vi "test-diff-drive-constraints.vi"() -> (3 "Test Passed":bool)   [LabVIEW 2019]
uses:
  <vilib>/Rock Robotics/WPI/ThirdParty/JAS_Junk/TrajLib/POSE2D.ctl
  <vilib>/Rock Robotics/WPI/ThirdParty/JAS_Junk/TrajLib/TRANSLATION2D.ctl
  <vilib>/Rock Robotics/WPI/ThirdParty/JAS_Junk/TrajLib/ROTATION2D.ctl
  <vilib>/Rock Robotics/SystemInterfaces/NetworkCommunication/NetComm_UsageReport_report.vi
  <vilib>/Rock Robotics/WPI/ThirdParty/JAS_Junk/TrajLib/DiffDriveKinematicsConstraint_New.vi
  <vilib>/Rock Robotics/WPI/ThirdParty/JAS_Junk/TrajLib/CentripetalAccelConstraint_New.vi
  <vilib>/Rock Robotics/WPI/ThirdParty/JAS_Junk/TrajLib/Util_LibraryGlobals.vi
  <vilib>/Rock Robotics/WPI/ThirdParty/JAS_Junk/TrajLib/Trajectory_Library.lvlib
panel:
  in  "Cent Feet Per Sec^2 2":dbl=12.0 format="%#_13g"
  out "Accel Exceeded":bool
  out "Acceleration":dbl[][](graph)
  out "Velocity":dbl[][](graph)
  out "Max Accel":dbl
  out "Max Ya":dbl
  out "max Xx":dbl
  in  "Feet/Sec":dbl=12.0 format="%#_13g"
  in  "Feet Per Sec^2":dbl=12.0 format="%#_13g"
  out "Max Speed":dbl
  out "Max Y vel":dbl
  out "max X vel":dbl
  out "XY Graph":cluster{dbl[], dbl[]}[](graph)
  out "Waypoints":T1[](array[typedef]) {"ROTATION"."SIN" format="%13.4f"; "ROTATION"."COS" format="%13.4f"; "ROTATION"."VALUE" format="%13.4f"; "TRANSLATION"."Y" format="%14.3f"; "TRANSLATION"."X" format="%14.3f"}
  out "TotalTImeSecs":dbl
  out "Speed Exceeded":bool
  out "error out":errorcluster
  # "9.1"
  # "5.7"
  # "9.55"
  # "6.59"
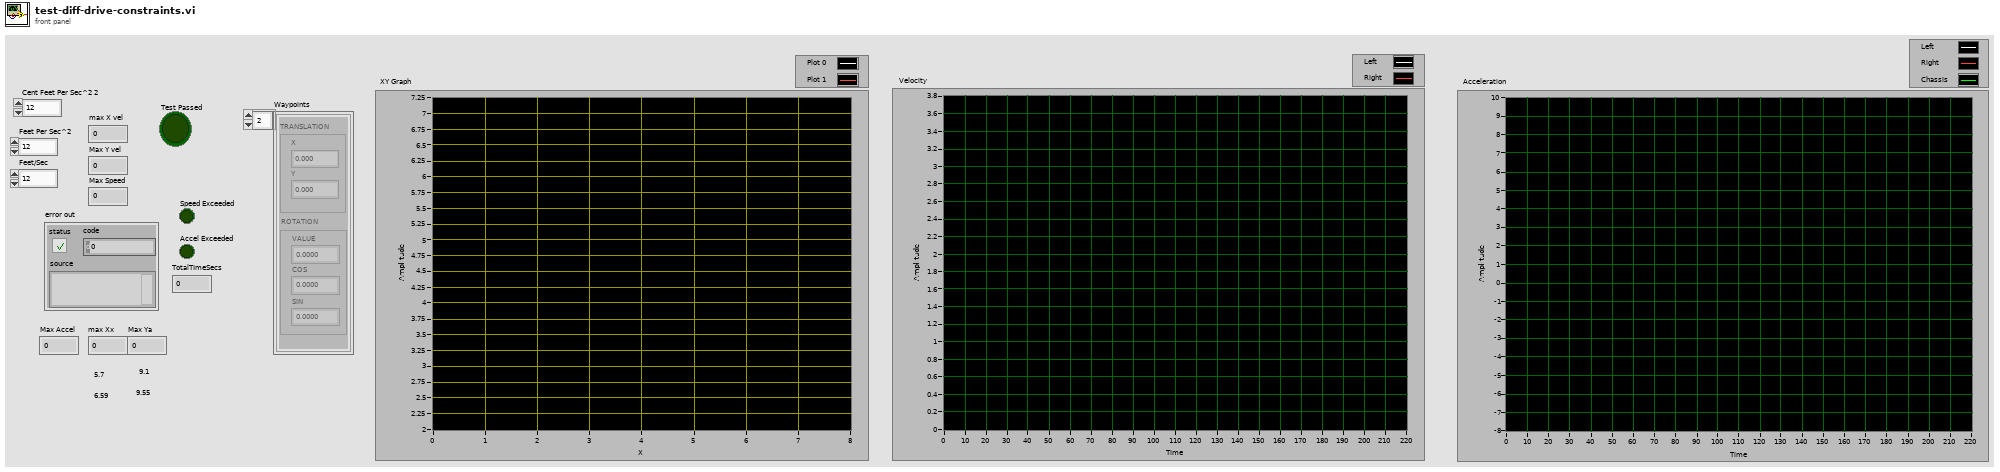
[diagram p1: front panel]
types:
  T1 = typedef "Trajectory_Library.lvlib/POSE2D.ctl" = cluster{"TRANSLATION":T2, "ROTATION":T3}
  T2 = typedef "Trajectory_Library.lvlib/TRANSLATION2D.ctl" = cluster{"X":dbl, "Y":dbl}
  T3 = typedef "Trajectory_Library.lvlib/ROTATION2D.ctl" = cluster{"VALUE":dbl, "COS":dbl, "SIN":dbl}
  T4 = typedef "Trajectory_Library.lvlib/DIFF_DRIVE_KINEMATICS.ctl" = cluster{"TrackWidth_Meters":dbl}
  T5 = typedef "Trajectory_Library.lvlib/TRAJ_CONFIG.ctl" = cluster{"MaxVelocity":dbl, "Max Acceleration":dbl, "StartVelocity":dbl, "End Velocity":dbl, "Reversed":bool, "DiffDrKineConstntDefined":bool, "CentAcellConstntDefined":bool, "DiffDrVoltConstntDefined":bool, "DIFF_DRIVE_KINE_CONSTRAINT":T6, "CENTRIPETAL_ACCEL_CONSTRAINT":T7, "SwerveDrKineConstntDefined":bool, "SWERVE_DRIVE_KINE_CONSTRAINT":T8, "DIFF_DRIVE_VOLTAGE_CONSTRAINT":T11, "MECANUM_DRIVE_KINE_CONSTRAINT":T13, "MecanumDrKineConstntDefined":bool}
  T6 = typedef "Trajectory_Library.lvlib/TRAJ_CONSTRAINT_DIIF_DRIVE_KINEMATICS.ctl" = cluster{"Max Speed (M/S)":dbl, "DIFF_DRIVE_KINEMATICS":T4, "Max Accel (M/S2)":dbl}
  T7 = typedef "Trajectory_Library.lvlib/TRAJ_CONSTRAINT_CENTRIPETAL_ACCEL.ctl" = cluster{"Max Cent Accel":dbl}
  T8 = typedef "Trajectory_Library.lvlib/TRAJ_CONSTRAINT_SWERVE_DRIVE_KINEMATICS.ctl" = cluster{"Max Speed (M/S)":dbl, "SwerveKinematics":T9}
  T9 = typedef "Trajectory_Library.lvlib/SWERVE_DRIVE_KINEMATICS.ctl" = cluster{"NumModules":i32, "InverseKinematics":T10, "ForwardKinematics":T10, "Modules":T2[], "PrevCoR":T2}
  T10 = typedef "NI_Matrix.lvlib/RealMatrix.ctl" = dbl[][]
  T11 = typedef "Trajectory_Library.lvlib/TRAJ_CONSTRAINT_DIIF_DRIVE_VOLTAGE.ctl" = cluster{"Max Voltage":dbl, "DIFF_DRIVE_KINEMATICS":T4, "SIMPLE_MOTOR_FF":T12}
  T12 = typedef "Trajectory_Library.lvlib/SIMPLE_MOTOR_FF.ctl" = cluster{"Ks":dbl, "Kv":dbl, "Ka":dbl}
  T13 = typedef "Trajectory_Library.lvlib/TRAJ_CONSTRAINT_MECA_DRIVE_KINEMATICS.ctl" = cluster{"Max Speed (M/S)":dbl, "MECA_DRIVE_KINEMATICS":T14}
  T14 = typedef "Trajectory_Library.lvlib/MECA_DRIVE_KINEMATICS.ctl" = cluster{"FrontLeft":T2, "FrontRight":T2, "RearLeft":T2, "RearRight":T2, "InverseKinematics":T10, "ForwardKinematics":T10, "PrevCoR":T2}
  T15 = typedef "Trajectory_Library.lvlib/TRAJECTORY.ctl" = cluster{"TotalTImeSecs":dbl, "States":T16[]}
  T16 = typedef "Trajectory_Library.lvlib/TRAJ_STATE.ctl" = cluster{"TimeSeconds":dbl, "Velocity":dbl, "Acceleration":dbl, "POSE":T1, "Curvature":dbl}
  T17 = typedef "Trajectory_Library.lvlib/CHASSIS_SPEEDS.ctl" = cluster{"vX":dbl, "vY":dbl, "vOmega":dbl}
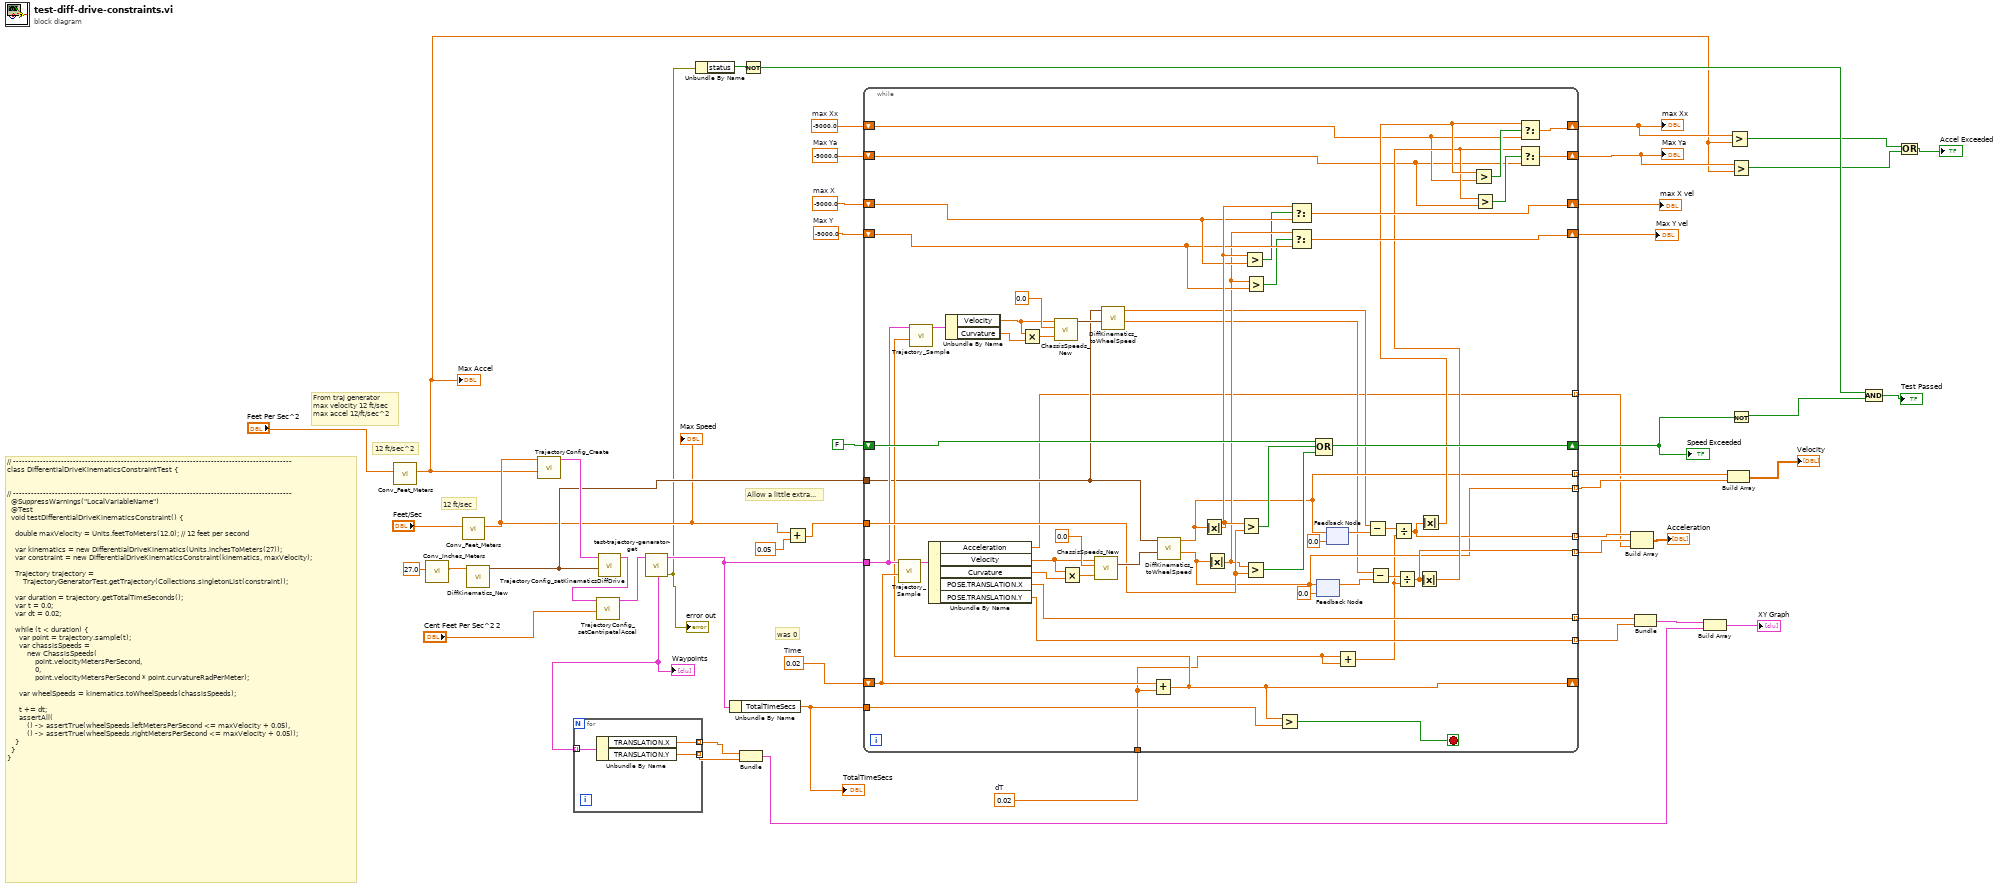
[diagram p0: block diagram]
diagram:
  w17 = -9000.0  # max Xx
  w18 = -9000.0  # Max Ya
  w27 = -9000.0  # max X
  w28 = -9000.0  # Max Y
  w43 = 0.02  # dT
  w45 = 0.02  # TIme
  # "was 0"
  # "Allow a little extra..."
  # "12 ft/sec^2"
  # "From traj generator\nmax velocity 12 ft/sec\nmax accel 12/ft/sec^2"
  # "12 ft/sec"
  # "// ---------------------------------------------------------------------------------------------\nclass DifferentialDriveKinematicsConstraintTest {\n\n\n// ---------------------------------------------------------------------------------------------\n  @SuppressWarnings(\"LocalVariableName\")\n  @Test\n  void testDifferentialDriveKinematicsConstraint() {\n\n    double maxVelocity = Units.feetToMeters(12.0); // 12 feet per second\n\n    var kinematics = new DifferentialDriveKinematics(Units.inchesToMeters(27));\n    var constraint = new DifferentialDriveKinematicsConstraint(kinematics, maxVelocity);\n\n    Trajectory trajectory =\n        TrajectoryGeneratorTest.getTrajectory(Collections.singletonList(constraint));\n\n    var duration = trajectory.getTotalTimeSeconds();\n    var t = 0.0;\n    var dt = 0.02;\n\n    while (t < duration) {\n      var point = trajectory.sample(t);\n      var chassisSpeeds =\n          new ChassisSpeeds(\n              point.velocityMetersPerSecond,\n              0,\n              point.velocityMetersPerSecond * point.curvatureRadPerMeter);\n\n      var wheelSpeeds = kinematics.toWheelSpeeds(chassisSpeeds);\n\n      t += dt;\n      assertAll(\n          () -> assertTrue(wheelSpeeds.leftMetersPerSecond <= maxVelocity + 0.05),\n          () -> assertTrue(wheelSpeeds.rightMetersPerSecond <= maxVelocity + 0.05));\n    }\n  }\n}"
  n1 = call <vilib>:"Conv_Feet_Meters.vi"("Feet"="Feet Per Sec^2") -> ("Meters"=w2:dbl)  [unwired: 10 in]
  "Max Accel" <- w2
  n2 = call <vilib>:"Conv_Inches_Meters.vi"("INCH"=27.0) -> ("Meters"=w50:dbl)  [unwired: 10 in]
  n3 = call <vilib>:"Conv_Feet_Meters.vi"("Feet"="Feet/Sec") -> ("Meters"=w39:dbl)  [unwired: 10 in]
  "Max Speed" <- w39
  n4 = call <vilib>:"DiffKinematics_New.vi"("TrackWidth_Meters"=w50) -> ("DIFF_DRIVE_KINEMATICS"=w41:T4)  [unwired: 10 in]
  n5 = call <vilib>:"TrajectoryConfig_Create.vi"("MaxAcceleration"=w2, "MaxVelocity"=w39) -> ("TRAJECTORY_CONFIG"=w47:T5)  [unwired: 9 in]
  n6 = call <vilib>:"TrajectoryConfig_setKinematicsDiffDrive.vi"("DIFF_DRIVE_KINEMATICS"=w41, "inTRAJECTORY_CONFIG"=w47) -> ("outTRAJECTORY_CONFIG"=w4:T5)  [unwired: 9 in]
  n7 = call <vilib>:"TrajectoryConfig_setCentripetalAccel.vi"("Max Cent Accel"="Cent Feet Per Sec^2 2", "inTRAJECTORY_CONFIG"=w4) -> ("outTRAJECTORY_CONFIG"=w3:T5)  [unwired: 9 in]
  n8 = call "test-trajectory-generator-get.vi"("traj_config"=w3) -> ("error out"=w21:errorcluster, "TRAJECTORY"=w42:T15, "Waypoints"=w36:T1[])  [unwired: 8 in]
  "error out" <- w21
  "Waypoints" <- w36
  n9 = for {
    tunnel: w36 -> [w53] mode=indexing
    tunnel: [w52] -> w35 mode=indexing
    tunnel: [w51] -> w34 mode=indexing
    n10 = Unbundle By Name(w53) -> ("TRANSLATION.X"=w52:dbl, "TRANSLATION.Y"=w51:dbl)
  }
  n11 = Unbundle By Name(w21) -> ("status"=w20:bool)
  n12 = Unbundle By Name(w42) -> ("TotalTImeSecs"=w44:dbl)
  "TotalTImeSecs" <- w44
  n13 = Bundle(w35, w34) -> (w30:cluster{dbl[], dbl[]})  [unwired: 1 in]
  n14 = Not(x=w20) -> (.not. x?=w19:bool)
  n15 = Add(x=w39, y=0.05) -> (x+y=w38:dbl)
  n16 = while {
    tunnel: w44 -> [w109]
    shift-right: [w66] -> _
    shift-left: w45 -> [w107]
    tunnel: w43 -> [w55]
    tunnel: w42 -> [w67]
    tunnel: w41 -> [w60]
    shift-right: [w99] -> w22
    shift-left: FALSE -> [w100]
    tunnel: w38 -> [w96]
    tunnel: [w95] -> w33 mode=indexing
    tunnel: [w94] -> w32 mode=indexing
    shift-right: [w92] -> w26
    shift-left: w27 -> [w90]
    shift-right: [w93] -> w25
    shift-left: w28 -> [w89]
    shift-right: [w73] -> w8
    shift-left: w17 -> [w75]
    shift-right: [w72] -> w7
    shift-left: w18 -> [w74]
    tunnel: [w71] -> w16 mode=indexing
    tunnel: [w58] -> w15 mode=indexing
    tunnel: [w70] -> w13 mode=indexing
    tunnel: [w69] -> w12 mode=indexing
    tunnel: [w54] -> w10 mode=indexing
    stop <- w108 stop-if-true
    n17 = call <vilib>:"Trajectory_Sample.vi"("Time"=w107, "InputTRAJECTORY"=w67) -> ("OutputTRAJ_STATE"=w106:T16)  [unwired: 9 in]
    n18 = Unbundle By Name(w106) -> ("Acceleration"=w54:dbl, "Velocity"=w103:dbl, "Curvature"=w102:dbl, "POSE.TRANSLATION.X"=w95:dbl, "POSE.TRANSLATION.Y"=w94:dbl)
    n19 = Multiply(x=w103, y=w102) -> (x*y=w104:dbl)
    n20 = call <vilib>:"ChassisSpeeds_New.vi"("vAngular"=w104, "vY"=0.0, "vX"=w103) -> ("CHASSIS"=w101:T17)  [unwired: 8 in]
    n21 = Add(x=w107, y=w55) -> (x+y=w66:dbl)
    n22 = call <vilib>:"Trajectory_Sample.vi"("Time"=w66, "InputTRAJECTORY"=w67) -> ("OutputTRAJ_STATE"=w68:T16)  [unwired: 9 in]
    n23 = Unbundle By Name(w68) -> ("Velocity"=w63:dbl, "Curvature"=w62:dbl)
    n24 = Multiply(x=w63, y=w62) -> (x*y=w64:dbl)
    n25 = call <vilib>:"ChassisSpeeds_New.vi"("vAngular"=w64, "vY"=0.0, "vX"=w63) -> ("CHASSIS"=w61:T17)  [unwired: 8 in]
    n26 = call <vilib>:"DiffKinematics_toWheelSpeed.vi"("CHASSIS Speed"=w61, "DIFF_DRIVE_KINEMATICS"=w60) -> ("RightVelocity"=w57:dbl, "LeftVelocity"=w59:dbl)  [unwired: 8 in]
    n27 = call <vilib>:"DiffKinematics_toWheelSpeed.vi"("CHASSIS Speed"=w101, "DIFF_DRIVE_KINEMATICS"=w60) -> ("RightVelocity"=w58:dbl, "LeftVelocity"=w71:dbl)  [unwired: 8 in]
    n28 = Absolute Value(x=w71) -> (abs(x)=w91:dbl)
    n29 = Absolute Value(x=w58) -> (abs(x)=w88:dbl)
    n30 = Greater?(x=w91, y=w96) -> (0:w98:bool)
    n31 = Greater?(x=w91, y=w90) -> (0:w87:bool)
    n32 = Greater?(x=w88, y=w96) -> (0:w97:bool)
    n33 = Greater?(x=w88, y=w89) -> (0:w86:bool)
    n34 = Greater?(x=w66, y=w109) -> (0:w108:bool)
    n35 = Select(t=w91, s=w87, f=w90) -> (s? t:f=w92:dbl)
    n36 = Select(t=w88, s=w86, f=w89) -> (s? t:f=w93:dbl)
    n37 = Compound Arithmetic op=OR(w100, w98, w97) -> (w99:bool)
    n38 = feedback #1(0.0 ("RightVelocity")) -> (w82:dbl)
    n39 = feedback-in #1(w58) -> ()
    n40 = feedback-in #2(w71) -> ()
    n41 = feedback #2(0.0 ("LeftVelocity")) -> (w83:dbl)
    n42 = Add(x=w55, y=w55) -> (x+y=w56:dbl)
    n43 = Subtract(x=w59, y=w83) -> (x-y=w81:dbl)
    n44 = Subtract(x=w57, y=w82) -> (x-y=w80:dbl)
    n45 = Divide(x=w81, y=w56) -> (x/y=w70:dbl)
    n46 = Divide(x=w80, y=w56) -> (x/y=w69:dbl)
    n47 = Absolute Value(x=w69) -> (abs(x)=w76:dbl)
    n48 = Absolute Value(x=w70) -> (abs(x)=w77:dbl)
    n49 = Greater?(x=w77, y=w75) -> (0:w79:bool)
    n50 = Greater?(x=w76, y=w74) -> (0:w78:bool)
    n51 = Select(t=w77, s=w79, f=w75) -> (s? t:f=w73:dbl)
    n52 = Select(t=w76, s=w78, f=w74) -> (s? t:f=w72:dbl)
  }
  "Speed Exceeded" <- w22
  "max X vel" <- w26
  "Max Y vel" <- w25
  "max Xx" <- w8
  "Max Ya" <- w7
  n53 = Build Array(w13, w12, w10) -> (→"Acceleration":dbl[][])
  n54 = Bundle(w33, w32) -> (w31:cluster{dbl[], dbl[]})  [unwired: 1 in]
  n55 = Build Array(w31, w30) -> (→"XY Graph":cluster{dbl[], dbl[]}[])
  n56 = Build Array(w16, w15) -> (→"Velocity":dbl[][])
  n57 = Greater?(x=w8, y=w2) -> (0:w6:bool)
  n58 = Greater?(x=w7, y=w2) -> (0:w5:bool)
  n59 = Not(x=w22) -> (.not. x?=w23:bool)
  n60 = Compound Arithmetic op=AND(w19, w23) -> (→"Test Passed":bool)
  n61 = Compound Arithmetic op=OR(w6, w5) -> (→"Accel Exceeded":bool)
